vi "swerve drive one remote.vi"(8 "spin":i32, 9 "move2":i32, 10 "move1":i32, 11 "JoystickDevRef":T2) -> (2 "output cluster":T1)   [LabVIEW 2019]
uses:
  <vilib>/Rock Robotics/WPI/Joystick/WPI_JoystickDevRef.ctl
  <vilib>/Rock Robotics/WPI/Joystick/WPI_JoystickDeviceEnum.ctl
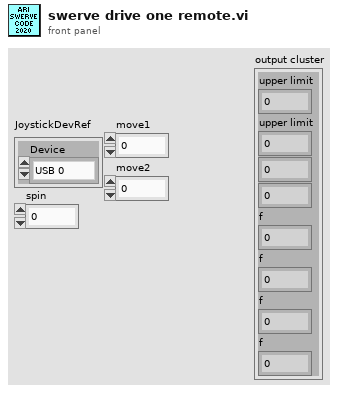
[diagram p1: front panel]
types:
  T1 = cluster{"upper limit":dbl, "upper limit":dbl, dbl, dbl, "f":dbl, "f":dbl, "f":dbl, "f":dbl}
  T2 = typedef "WPI_JoystickDevRef.ctl" = cluster{"Device":T3}
  T3 = typedef "WPI_JoystickDeviceEnum.ctl" = enum16{"USB 0", "USB 1", "USB 2", "USB 3", "USB 4", "USB 5"}
  T4 = cluster{"upper limit":dbl, dbl, "upper limit":dbl, dbl, dbl, dbl, dbl, dbl}
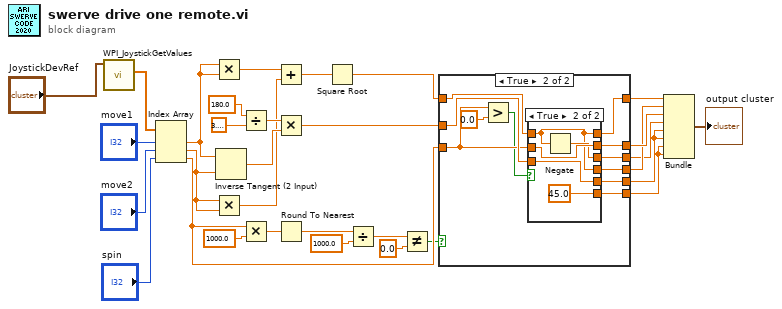
[diagram p0: block diagram]
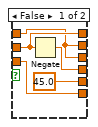
[diagram p3: hidden frame]
diagram:
  n1 = call <vilib>:"WPI_JoystickGetValues.vi"("JoystickDevRef"="JoystickDevRef") -> ("Axes"=w30:dbl[])  [unwired: 6 in, 4 out]
  n2 = Index Array(array=w30, index #1="move1", index #2="move2", index #3="spin") -> (element #1=w22:dbl, element #2=w21:dbl, element #3=w5:dbl)
  n3 = Multiply(x=w22, y=w22) -> (x*y=w20:dbl)
  n4 = Multiply(x=w21, y=w21) -> (x*y=w19:dbl)
  n5 = Inverse Tangent (2 Input)(1:w21, 2:w22) -> (0:w23:dbl)
  n6 = Divide(x=180.0, y=3.141592653589793) -> (x/y=w24:dbl)
  n7 = Multiply(x=w5, y=1000.0) -> (x*y=w8:dbl)
  n8 = Add(x=w20, y=w19) -> (x+y=w18:dbl)
  n9 = Multiply(x=w24, y=w23) -> (x*y=w15:dbl)
  n10 = Round To Nearest(number=w8) -> (nearest integer value=w7:dbl)
  n11 = Square Root(x=w18) -> (sqrt(x)=w16:dbl)
  n12 = Divide(x=w7, y=1000.0) -> (x/y=w3:dbl)
  n13 = Not Equal?(x=w3, y=0.0) -> (x != y?=w2:bool)
  n14 = case shown="True" w2 {
    tunnel: [w33 w44] -> w17
    tunnel: w16 -> [w32 w43]
    tunnel: w15 -> [w33 w42]
    tunnel: [w33 w41] -> w14
    tunnel: [w32 w40] -> w13
    tunnel: w5 -> [_ w36]
    tunnel: [w32 w39] -> w12
    tunnel: [w32 w38] -> w11
    tunnel: [w32 w37] -> w10
    frame False {
    }
    frame True {
      n15 = Greater?(x=w36, y=0.0) -> (0:w35:bool)
      n16 = case shown="True" w35 {
        tunnel: [w48 45.0] -> w44
        tunnel: w43 -> [w45 w50]
        tunnel: [45.0 w53] -> w41
        tunnel: w42 -> [w48 w53]
        tunnel: [w47 w50] -> w40
        tunnel: [w45 w52] -> w39
        tunnel: w36 -> [w47 w52]
        tunnel: [w46 w50] -> w38
        tunnel: [w45 w51] -> w37
        frame False {
          n17 = Negate(x=w47) -> (-x=w46:dbl)
        }
        frame True {
          n18 = Negate(x=w50) -> (-x=w51:dbl)
        }
      }
    }
  }
  n19 = Bundle("upper limit"=w13, w11, "upper limit"=w12, w10, w14, w14, w17, w17) -> (→"output cluster":T4)  [unwired: 1 in]
